vi "Read LV Type Attrs.vi"(8 "error in (no error)":errorcluster, 11 "LVType Ref":T3) -> (0 "error out":errorcluster, 1 "Type Descriptor":i16[](array[numeric]), 2 "Type Name":string, 3 "LVType Ref out":T3, 5 "Unit String":string, 7 "Units":T1[](array[typedef]))   [LabVIEW 2017]
uses:
  <vilib>/UPVI/lvhdf5/library.llb/HDF5 Ref.ctl
  <vilib>/Utility/VariantDataType/UnitInfo.ctl
  <vilib>/Utility/VariantDataType/UnitType.ctl
  <vilib>/Utility/VariantDataType/VariantType.lvlib
panel:
  # "LVHDF5 Toolkit\nCopyright (c) 2005-2013 by Jason D. Sommerville\nCopyright (c) 2014 by UPVI, LLC.\n\nThis use and distribution of this file is governed by the terms found in \nLICENSE.txt distributed with this toolkit and installed at\n <user.lib>\\_lvhdf5\\LICENSE.txt"
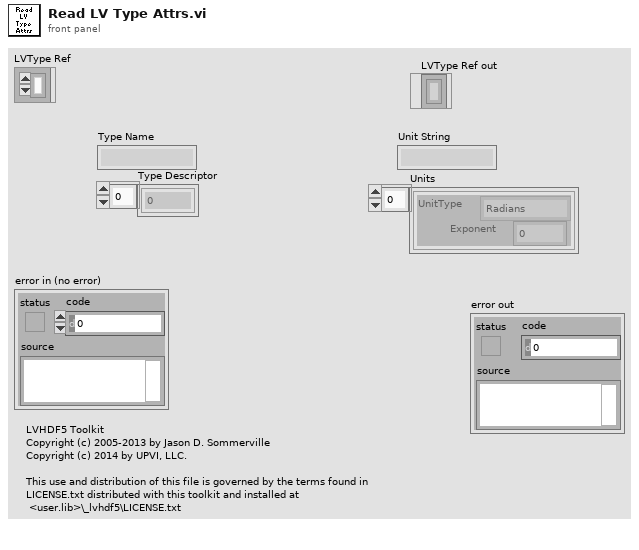
[diagram p1: front panel]
types:
  T1 = typedef "VariantType.lvlib/UnitInfo.ctl" = cluster{"UnitType":T2, "Exponent":i16}
  T2 = typedef "VariantType.lvlib/UnitType.ctl" = enum16{"Radians", "Steradians", "Seconds", "Meters", "Kilograms", "Amperes", "Kelvins", "Moles", "Candelas", "InvalidUnit"}
  T3 = typedef "HDF5 Ref.ctl" = refnum<k1>
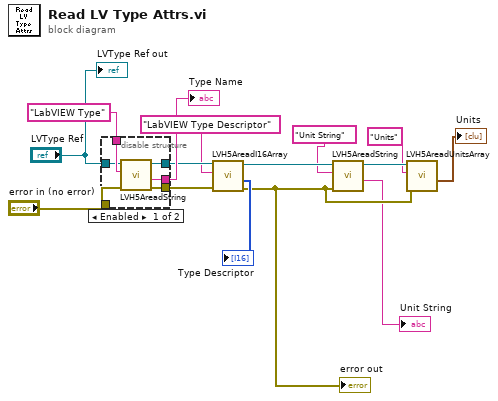
[diagram p0: block diagram]
diagram:
  n1 = disable-structure shown="Enabled" {
    disable-tunnel: "LabVIEW Type" -> [w21 _]
    disable-tunnel: "LVType Ref" -> [w20 w23]
    disable-tunnel: "error in (no error)" -> [w19 w22]
    disable-tunnel: [w18 _] -> w12
    disable-tunnel: [w17 w22] -> w11
    disable-tunnel: [w16 w23] -> w10
    frame Enabled {
      n2 = call <vilib>:"LVH5AreadString.vi"("error in (no error)"=w19, "Name"=w21, "HDF5 Location in"=w20) -> ("error out"=w17:errorcluster, "Value"=w18:string, "HDF5 Location out"=w16:T3)  [unwired: 4 in]
    }
    frame Disabled {
    }
  }
  "Type Name" <- w12
  n3 = call <vilib>:"LVH5AreadI16Array.vi"("error in (no error)"=w11, "Name"="LabVIEW Type Descriptor", "HDF5 Location in"=w10) -> ("error out"=w6:errorcluster, "Value"=→"Type Descriptor":i16[], "HDF5 Location out"=w7:T3)  [unwired: 4 in]
  "error out" <- w6
  n4 = call <vilib>:"LVH5AreadString.vi"("error in (no error)"=w6, "Name"="Unit String", "HDF5 Location in"=w7) -> ("Value"=→"Unit String":string, "HDF5 Location out"=w3:T3)  [unwired: 4 in, 1 out]
  n5 = call <vilib>:"LVH5AreadUnitsArray.vi"("error in (no error)"=w6, "Name"="Units", "HDF5 Location in"=w3) -> ("Value"=→"Units":T1[])  [unwired: 4 in, 2 out]
  "LVType Ref out" <- "LVType Ref"
